vi "STOP.vi"(8 "error in (no error)":errorcluster, 11 "Stop in":refnum<class "DB_SQLite.lvclass">) -> (0 "error out":errorcluster, 3 "Stop out":refnum<class "DB_SQLite.lvclass">)   [LabVIEW 2015, in "DB_SQLite.lvclass"]
uses:
  DB_SQLite.lvclass
  DB.lvclass
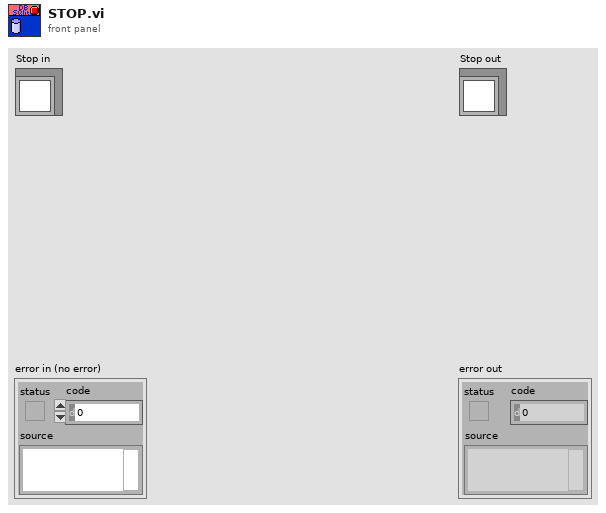
[diagram p1: front panel]
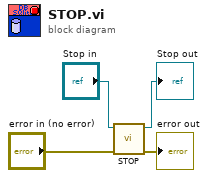
[diagram p0: block diagram]
diagram:
  n1 = call-parent "STOP.vi"("error in (no error)"="error in (no error)", "Stop in"="Stop in") -> ("error out"=→"error out":errorcluster, "Stop out"=→"Stop out":refnum<class "DB_SQLite.lvclass">)  [unwired: 8 in]
